vi "rs-trigger.vi"(2 "S":bool, 3 "R":bool) -> (0 "notQ":bool, 1 "Q":bool)   [LabVIEW 2013]
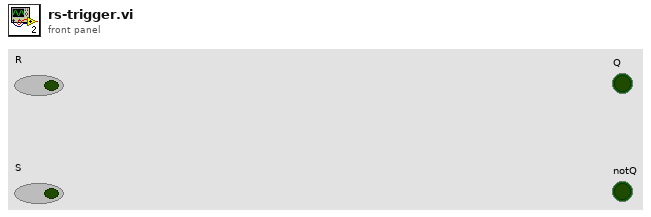
[diagram p1: front panel]
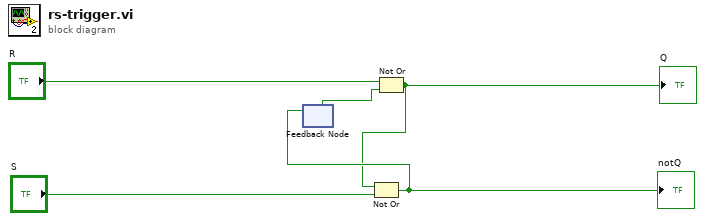
[diagram p0: block diagram]
diagram:
  n1 = feedback #1() -> (w5:bool)  [unwired: 1 in]
  n2 = Not Or(1:w5, 2:"R") -> (0:w3:bool)
  "Q" <- w3
  n3 = Not Or(1:"S", 2:w3) -> (0:w4:bool)
  "notQ" <- w4
  n4 = feedback-in #1(w4) -> ()
